vi "write_sample_parameters.vi"(3 "Parameters":T1, 8 "Error In":errorcluster, 10 "Sample":string, 11 "File Path":path) -> (0 "Error Out":errorcluster)   [LabVIEW 2019]
uses:
  parameters_cluster_typedef.ctl
  <vilib>/Utility/config.llb/Write Key (Double).vi
  <vilib>/Utility/config.llb/NI_LVConfig.lvlib
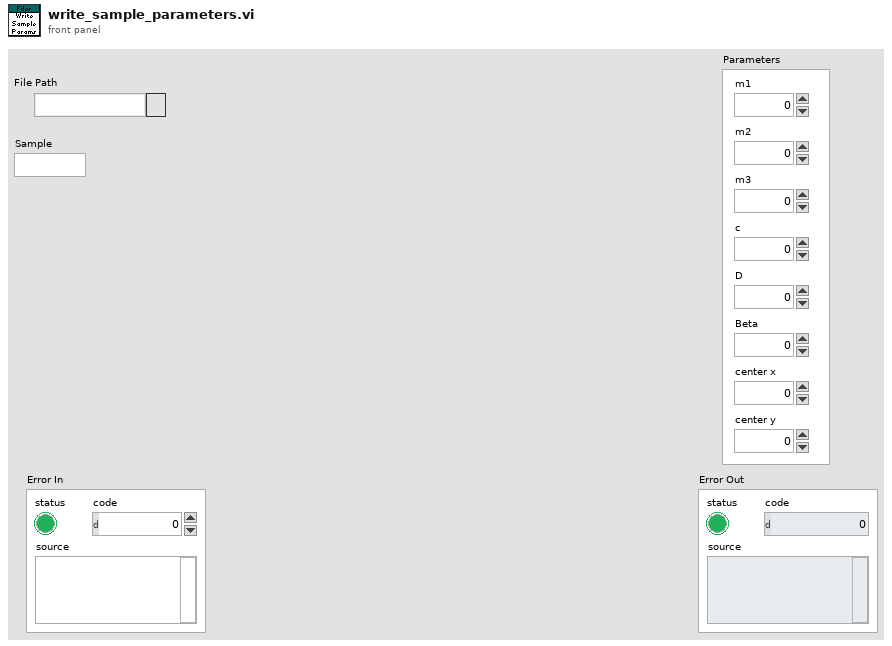
[diagram p1: front panel]
types:
  T1 = typedef "parameters_cluster_typedef.ctl" = cluster{"m1":dbl, "m2":dbl, "m3":dbl, "c":dbl, "D":dbl, "Beta":dbl, "center x":dbl, "center y":dbl}
  T2 = typedef "NI_LVConfig.lvlib/Config Data RefNum.ctl" = refnum<k1>
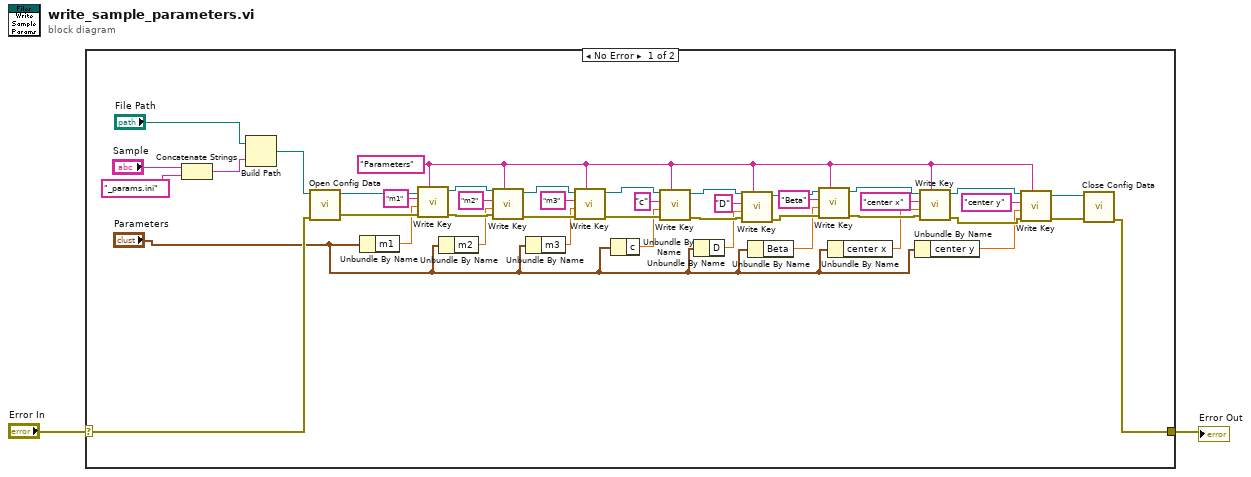
[diagram p0: block diagram]
diagram:
  n1 = case shown="No Error" "Error In" {
    selector: "Error In" -> [w40 w46]
    tunnel: [w3 w46] -> w1
    frame No Error {
      w28 = "Parameters" ("section")
      n2 = Concatenate Strings("Sample", "_params.ini" ("string")) -> (w42:string)
      n3 = Build Path(base path="File Path", name or relative path=w42) -> (appended path=w41:path)
      n4 = call <vilib>:"Open Config Data.vi"("error in (no error)"=w40, "configuration file path"=w41) -> ("error out"=w38:errorcluster, "refnum"=w39:T2)  [unwired: 7 in, 1 out]
      n5 = Unbundle By Name("Parameters") -> ("m1"=w36:dbl)
      n6 = call-poly <vilib>:"Write Key.vi"("section"=w28, "error in (no error)"=w38, "value"=w36, "key"="m1", "refnum"=w39) -> ("error out"=w27:errorcluster, "refnum out"=w14:T2)  [unwired: 4 in, 1 out]
      n7 = Unbundle By Name("Parameters") -> ("m2"=w13:dbl)
      n8 = call-poly <vilib>:"Write Key.vi"("section"=w28, "error in (no error)"=w27, "value"=w13, "key"="m2", "refnum"=w14) -> ("error out"=w26:errorcluster, "refnum out"=w20:T2)  [unwired: 4 in, 1 out]
      n9 = Unbundle By Name("Parameters") -> ("m3"=w12:dbl)
      n10 = call-poly <vilib>:"Write Key.vi"("section"=w28, "error in (no error)"=w26, "value"=w12, "key"="m3", "refnum"=w20) -> ("error out"=w25:errorcluster, "refnum out"=w19:T2)  [unwired: 4 in, 1 out]
      n11 = Unbundle By Name("Parameters") -> ("c"=w11:dbl)
      n12 = call-poly <vilib>:"Write Key.vi"("section"=w28, "error in (no error)"=w25, "value"=w11, "key"="c", "refnum"=w19) -> ("error out"=w24:errorcluster, "refnum out"=w18:T2)  [unwired: 4 in, 1 out]
      n13 = Unbundle By Name("Parameters") -> ("D"=w10:dbl)
      n14 = call-poly <vilib>:"Write Key.vi"("section"=w28, "error in (no error)"=w24, "value"=w10, "key"="D", "refnum"=w18) -> ("error out"=w23:errorcluster, "refnum out"=w17:T2)  [unwired: 4 in, 1 out]
      n15 = Unbundle By Name("Parameters") -> ("Beta"=w9:dbl)
      n16 = call-poly <vilib>:"Write Key.vi"("section"=w28, "error in (no error)"=w23, "value"=w9, "key"="Beta", "refnum"=w17) -> ("error out"=w22:errorcluster, "refnum out"=w16:T2)  [unwired: 4 in, 1 out]
      n17 = Unbundle By Name("Parameters") -> ("center x"=w8:dbl)
      n18 = Unbundle By Name("Parameters") -> ("center y"=w6:dbl)
      n19 = call-poly <vilib>:"Write Key.vi"("section"=w28, "error in (no error)"=w22, "value"=w8, "key"="center x", "refnum"=w16) -> ("error out"=w21:errorcluster, "refnum out"=w15:T2)  [unwired: 4 in, 1 out]
      n20 = call-poly <vilib>:"Write Key.vi"("section"=w28, "error in (no error)"=w21, "value"=w6, "key"="center y", "refnum"=w15) -> ("error out"=w4:errorcluster, "refnum out"=w5:T2)  [unwired: 4 in, 1 out]
      n21 = call <vilib>:"Close Config Data.vi"("error in (no error)"=w4, "refnum"=w5) -> ("error out"=w3:errorcluster)  [unwired: 8 in, 1 out]
    }
    frame Error {
    }
  }
  "Error Out" <- w1
